vi "Write to DB_12042024.vi"(8 "error in (no error)":errorcluster, 11 "Database Entry in":refnum<class "Database Entry.lvclass">) -> (0 "error out":errorcluster, 2 "Stack names":string[](array[string]), 3 "Database Entry out":refnum<class "Database Entry.lvclass">)   [LabVIEW 2021, in "Database Entry.lvclass"]
uses:
  Database Entry.lvclass
  Database Entry.lvclass/Database Entry.ctl
  <vilib>/Utility/file.llb/Read Delimited Spreadsheet (string).vi
  <vilib>/Utility/file.llb/Write Delimited Spreadsheet (string).vi
  Components/Stack/Stack.lvclass
panel:
  out "Final name":string
  out "Data cluster":T1={"module or proto"="proto", " geometry"="full", "resolution"="LD", "baselayer"="BA_123", "toplayer"="SI_789", "bl_pos"="1", "tl_pos"="1", "put_pos"="1", "region"="1", "asstray"="1", "comptray"="1", "put"="1", "date"="2024-04-02", "timestart"="1:12:12.442", "timeend"="1:23:45.244", "operator"="cmuperson", "tape"="some", "glue"="some", "stack name"="some", "Adhesive type"="", "Comments"="", "Temperature"="", "Relative Humidity"=""}
  out "error out py":errorcluster
  out "String Out":string="Upload Success"
  in  "error in (no error) py":errorcluster
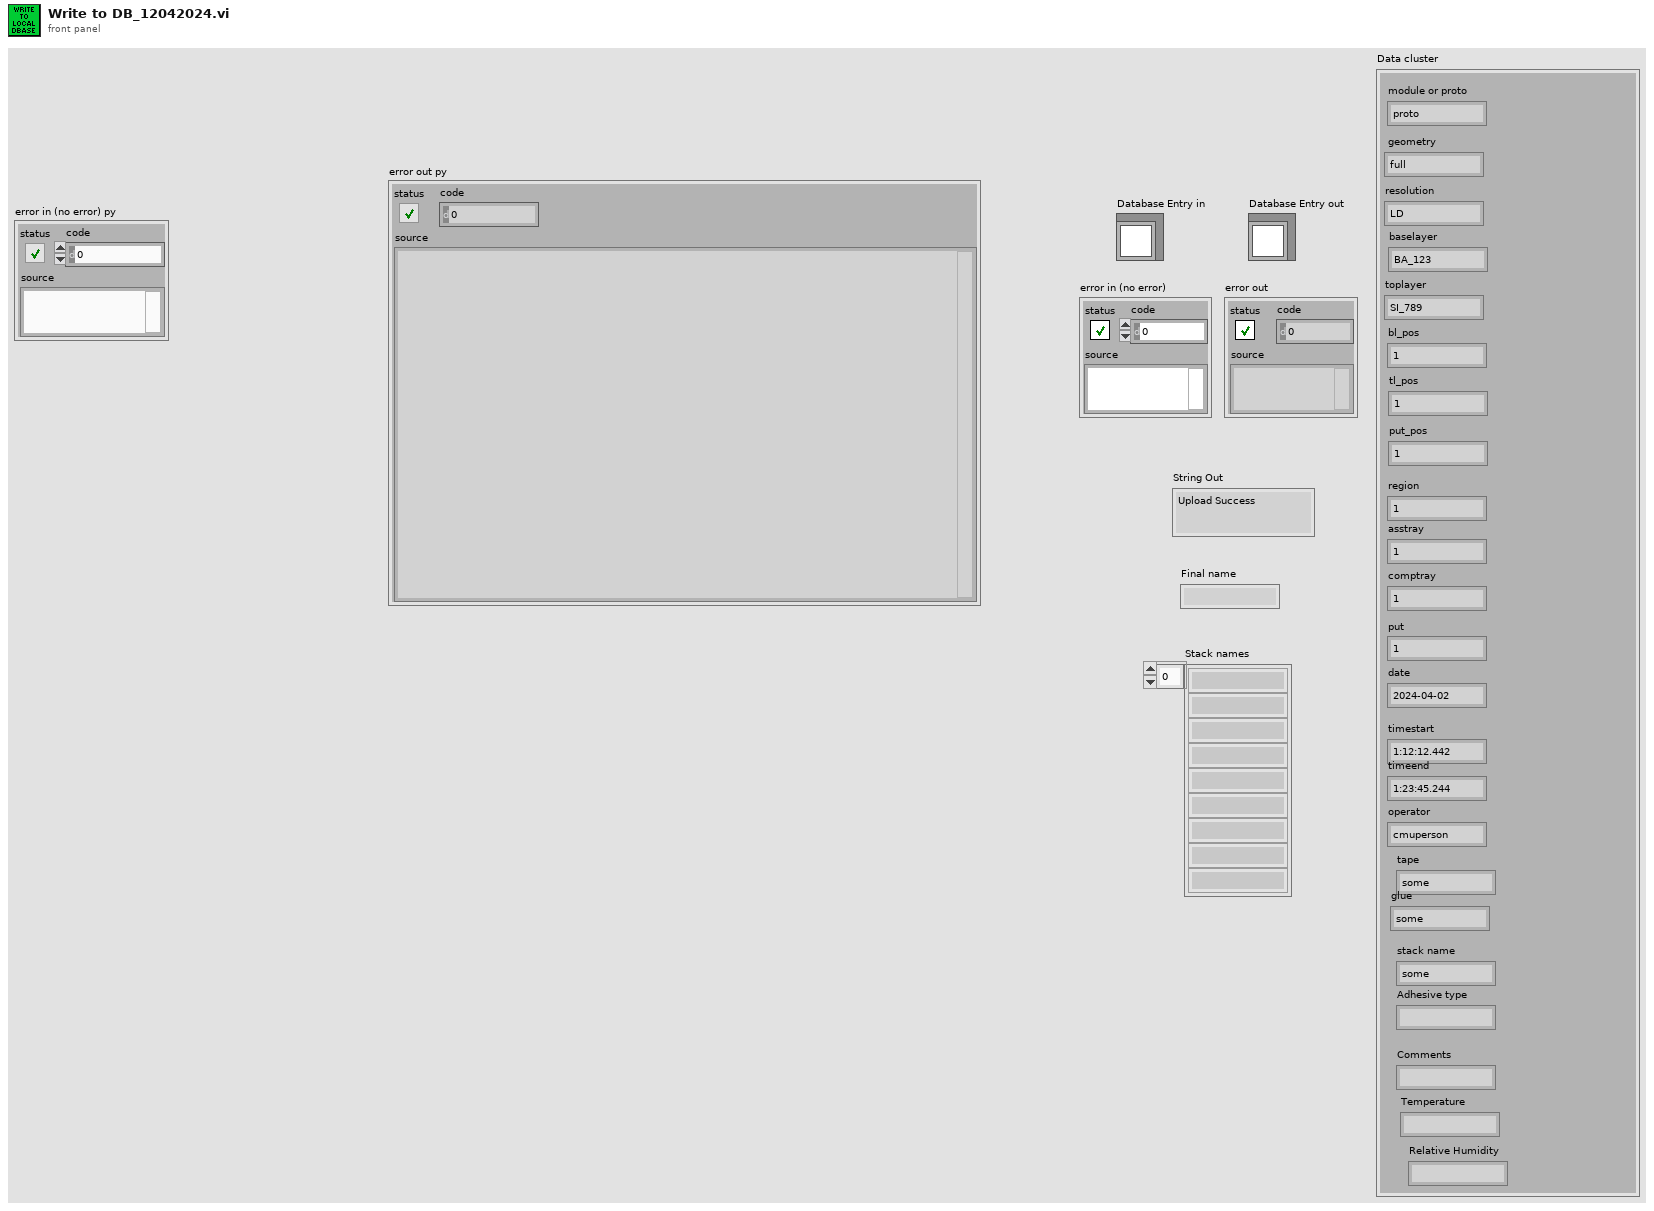
[diagram p1: front panel]
types:
  T1 = cluster{"module or proto":string, " geometry":string, "resolution":string, "baselayer":string, "toplayer":string, "bl_pos":string, "tl_pos":string, "put_pos":string, "region":string, "asstray":string, "comptray":string, "put":string, "date":string, "timestart":string, "timeend":string, "operator":string, "tape":string, "glue":string, "stack name":string, "Adhesive type":string, "Comments":string, "Temperature":string, "Relative Humidity":string}
  T2 = typedef "File Paths.ctl" = cluster{"Glue Pattern Folder":path, "Carrier Tray Folder":path, "Pick Up Tool Fixture Folder":path, "Components Folder":path, "Bellows Tool Offset.txt":path, "Pick Up Tool Offset.txt":path, "Dispense Tip Offset.txt":path, "Log Files":path, "Gantry Assembly Map.txt":path, "Syringe and offset map.txt":path, "Controllers Folder":path, "Local dbase config":path}
  T3 = cluster{"type":string, " geometry":string, "resolution":string, "baselayer":string, "toplayer":string, "bl_pos":string, "tl_pos":string, "put_pos":string, "region":string, "asstray":string, "comptray":string, "put":string, "date":string, "timestart":string, "timeend":string, "operator":string, "tape":string, "glue":string, "stack name":string, "Adhesive type":string, "Comments":string, "Temperature":string, "Relative Humidity":string}
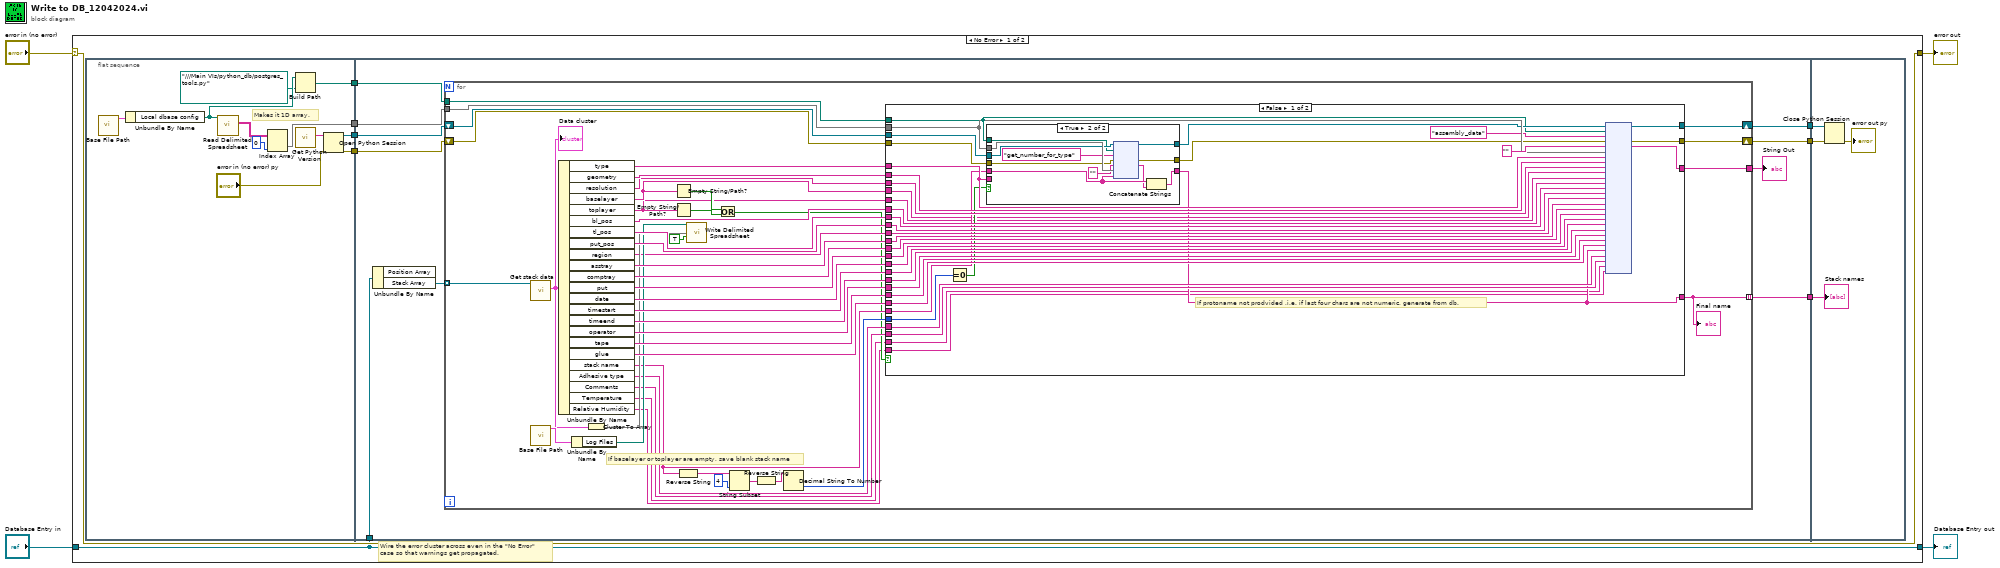
[diagram p0: block diagram]
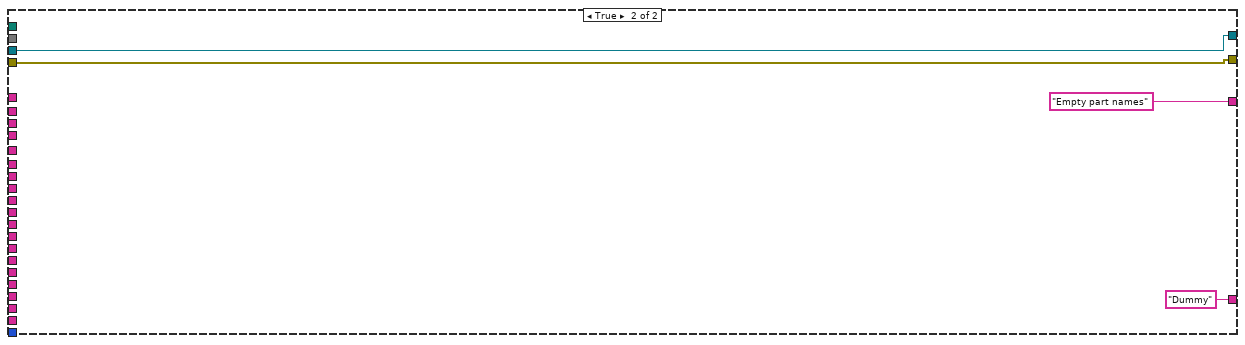
[diagram p3: hidden frame]
diagram:
  n1 = case shown="No Error" "error in (no error)" {
    selector: "error in (no error)" -> [w13 w140]
    tunnel: [w13 w140] -> w3
    tunnel: [w6 w139] -> w1
    tunnel: "Database Entry in" -> [w6 w139]
    frame No Error {
      # "Wire the error cluster across even in the \"No Error\"\ncase so that warnings get propagated."
      n2 = flat-sequence {
        tunnel: [w23] -> w12
        tunnel: [w24] -> w11
        tunnel: [w20] -> w10
        tunnel: [w16] -> w9
        tunnel: [w33] -> w8
        tunnel: [w32] -> w7
        tunnel: w12 -> [w34]
        tunnel: w11 -> [w31]
        tunnel: w10 -> [w30]
        tunnel: w9 -> [w29]
        tunnel: w6 -> [w28]
        tunnel: [w25] -> w5
        tunnel: w8 -> [w137]
        tunnel: w7 -> [w138]
        tunnel: w5 -> [w135]
        frame #0 {
          # "Makes it 1D array."
          n3 = call "Base File Path.vi"() -> ("Paths Out"=w21:T2)  [unwired: 11 in]
          n4 = Unbundle By Name(w21) -> ("Local dbase config"=w19:path)
          n5 = call-poly <vilib>:"Read Delimited Spreadsheet.vi"("file path (dialog if empty)"=w19) -> ("all rows"=w18:string[][])  [unwired: 9 in, 5 out]
          n6 = Index Array(array=w18, index (col)=0 ("disabled index (col)")) -> (element=w16:string[])  [unwired: 1 in]
          n7 = Build Path(base path=w19, name or relative path=path "../../../Main VIs/python_db/postgres_tools.py" ("module path")) -> (appended path=w20:path)
          n8 = call "Get Python Version.vi"() -> ("Python Version"=w14:string)  [unwired: 10 in, 1 out]
          n9 = Open Python Session(python version=w14, 3:"error in (no error) py") -> (session out=w24:refnum<k35>, error out=w23:errorcluster)  [unwired: 1 in]
        }
        frame #1 {
          n10 = Unbundle By Name(w28) -> ("Stack Array"=w26:refnum<class "Stack.lvclass">[])  [unwired: 1 out]
          n11 = for {
            tunnel: w30 -> [w54]
            shift-right: [w79] -> w33
            shift-left: w34 -> [w53]
            shift-right: [w78] -> w32
            shift-left: w31 -> [w55]
            tunnel: [w77] -> w27
            tunnel: w26 -> [w76] mode=indexing
            tunnel: w29 -> [w56]
            tunnel: [w38] -> w25 mode=indexing
            # "If baselayer or toplayer are empty, save blank stack name"
            n12 = call "Get stack data.vi"("Stack in"=w76) -> ("Data cluster"=w50:T3)  [unwired: 8 in, 2 out]
            "Data cluster" <- w50
            n13 = call "Base File Path.vi"() -> ("Paths Out"=w59:T2)  [unwired: 11 in]
            n14 = Unbundle By Name(w50) -> ("type"=w57:string, "geometry"=w75:string, "resolution"=w74:string, "baselayer"=w42:string, "toplayer"=w40:string, "bl_pos"=w73:string, "tl_pos"=w72:string, "put_pos"=w71:string, "region"=w52:string, "asstray"=w70:string, "comptray"=w69:string, "put"=w68:string, "date"=w67:string, "timestart"=w66:string, "timeend"=w65:string, "operator"=w64:string, "tape"=w63:string, "glue"=w62:string, "stack name"=w43:string, "Adhesive type"=w51:string, "Comments"=w49:string, "Temperature"=w36:string, "Relative Humidity"=w35:string)
            n15 = Unbundle By Name(w59) -> ("Log Files"=w58:path)
            n16 = Cluster To Array(cluster=w50) -> (array=w61:string[])
            n17 = Empty String/Path?(string/path=w42) -> (empty?=w41:bool)
            n18 = Empty String/Path?(string/path=w40) -> (empty?=w39:bool)
            n19 = Reverse String(1:w43) -> (0:w48:string)
            n20 = call-poly <vilib>:"Write Delimited Spreadsheet.vi"("file path (dialog if empty)"=w58, "1D data"=w61, "append to file? (new file:F)"=TRUE) -> ()  [unwired: 11 in, 2 out]
            n21 = Or(x=w41, y=w39) -> (x .or. y?=w37:bool)
            n22 = String Subset(string=w48, length (rest)=4 ("length (rest)")) -> (substring=w46:string)  [unwired: 1 in]
            n23 = Reverse String(1:w46) -> (0:w45:string)
            n24 = Decimal String To Number(string=w45) -> (number=w44:i32)  [unwired: 2 in, 1 out]
            n25 = case shown="False" w37 {
              tunnel: [w116 w133] -> w79
              tunnel: [w115 w134] -> w78
              tunnel: [w114 "Empty part names"] -> w77
              tunnel: w75 -> [w112 _]
              tunnel: w74 -> [w111 _]
              tunnel: w73 -> [w110 _]
              tunnel: w72 -> [w109 _]
              tunnel: w71 -> [w108 _]
              tunnel: w70 -> [w107 _]
              tunnel: w69 -> [w106 _]
              tunnel: w68 -> [w105 _]
              tunnel: w67 -> [w104 _]
              tunnel: w66 -> [w103 _]
              tunnel: w65 -> [w102 _]
              tunnel: w64 -> [w101 _]
              tunnel: w63 -> [w100 _]
              tunnel: w62 -> [w99 _]
              tunnel: w57 -> [w98 _]
              tunnel: w56 -> [w97 _]
              tunnel: w55 -> [w96 w134]
              tunnel: w54 -> [w94 _]
              tunnel: w53 -> [w93 w133]
              tunnel: w52 -> [w90 _]
              tunnel: w51 -> [w89 _]
              tunnel: w49 -> [w88 _]
              tunnel: w44 -> [w87 _]
              tunnel: w43 -> [w86 _]
              tunnel: w42 -> [w84 _]
              tunnel: w40 -> [w83 _]
              tunnel: [w82 "Dummy" ("stack name")] -> w38
              tunnel: w36 -> [w81 _]
              tunnel: w35 -> [w80 _]
              frame False {
                # "If protoname not prodvided ,i.e. if last four chars are not numeric, generate from db."
                n26 = Equal To 0?(x=w87) -> (x = 0?=w85:bool)
                n27 = case shown="True" w85 {
                  tunnel: w98 -> [_ _]
                  tunnel: w86 -> [w117 w130]
                  tunnel: w97 -> [_ w129]
                  tunnel: w96 -> [w119 w128]
                  tunnel: [w119 w127] -> w95
                  tunnel: w94 -> [_ w126]
                  tunnel: w93 -> [w118 w125]
                  tunnel: [w118 w124] -> w92
                  tunnel: [w117 w123] -> w82
                  frame False {
                  }
                  frame True {
                    n28 = node(w128, w126, "get_number_for_type" ("function name"), w125, "" ("function name"), w129, w130) -> (w127:refnum<k35>, w124:errorcluster, w120:string)  [unwired: 2 in, 2 out]
                    n29 = Concatenate Strings(w130, w120) -> (w123:string)
                  }
                }
                n30 = node(w95, w94, "assembly_data" ("function name"), w92, "", w97, w98, w112, w111, w84, w83, w110, w109, w108, w90, w107, w106, w105, w104, w103, w102, w101, w100, w99, w82, w89, w88, w81, w80) -> (w115:refnum<k35>, w116:errorcluster, w114:string)  [unwired: 24 in, 2 out]
              }
              frame True {
              }
            }
            "Final name" <- w38
          }
          "String Out" <- w27
        }
        frame #2 {
          n31 = Close Python Session(session in=w138, error in=w137) -> (11:→"error out py":errorcluster)
          "Stack names" <- w135
        }
      }
    }
    frame Error {
    }
  }
  "error out" <- w3
  "Database Entry out" <- w1
